vi "Module Running as Singleton--error.vi"() -> (0 "error out":errorcluster)   [LabVIEW 2017, in "My Cloneable Module.lvlib"]
doc: "Outputs an error cluster containing a custom error code indicating the module was running as a singleton, but Start Module has the 'Run as Singleton' input set to FALSE.\n_____\nBased on Delacor QMH Project Template 3.1.0.34."
uses:
  My Cloneable Module.lvlib
  <vilib>/Utility/error.llb/Error Cluster From Error Code.vi
  <vilib>/ErrorRing/Error Ring.xnode
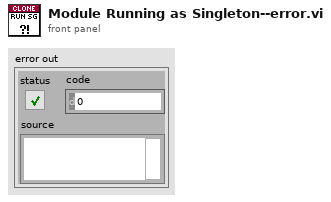
[diagram p1: front panel]
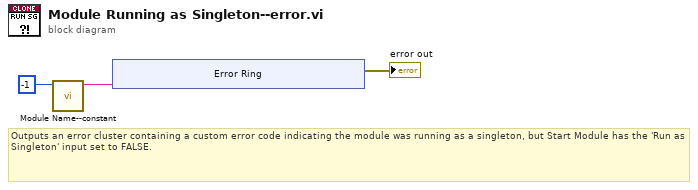
[diagram p0: block diagram]
diagram:
  # "Outputs an error cluster containing a custom error code indicating the module was running as a singleton, but Start Module has the 'Run as Singleton' input set to FALSE."
  n1 = call "Module Name--constant.vi"("Module ID"=-1) -> ("Module Name"=w3:string)  [unwired: 10 in]
  n2 = xnode "Error Ring"("parameter 0"=w3) -> ("error out"=→"error out":errorcluster)
